vi "EstimateHeuristicCost.vi"(9 "Goal":dbl[](array[numeric]), 10 "Nó atual":dbl[](array[numeric]), 11 "GridParameter":dbl) -> (2 "Heuristic":dbl)   [LabVIEW 2016]
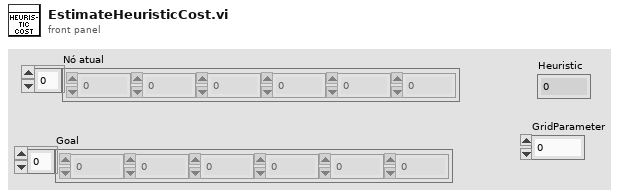
[diagram p1: front panel]
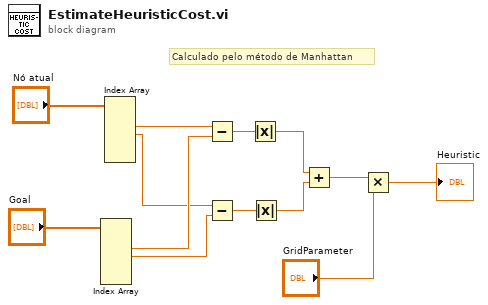
[diagram p0: block diagram]
diagram:
  # "Calculado pelo método de Manhattan"
  n1 = Index Array(array="Goal") -> (element #2=w10:dbl, element #3=w6:dbl)  [unwired: 6 in, 4 out]
  n2 = Index Array(array="Nó atual") -> (element #2=w11:dbl, element #3=w7:dbl)  [unwired: 6 in, 4 out]
  n3 = Subtract(x=w11, y=w10) -> (x-y=w9:dbl)
  n4 = Subtract(x=w7, y=w6) -> (x-y=w5:dbl)
  n5 = Absolute Value(x=w9) -> (abs(x)=w8:dbl)
  n6 = Absolute Value(x=w5) -> (abs(x)=w4:dbl)
  n7 = Add(x=w8, y=w4) -> (x+y=w3:dbl)
  n8 = Multiply(x=w3, y="GridParameter") -> (x*y=→"Heuristic":dbl)
